vi "CreatingandAccessingFiles.vi"() -> ()   [LabVIEW 2020]
panel:
  out "appended path":path
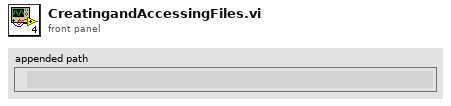
[diagram p1: front panel]
types:
  T1 = enum16{"open", "replace", "create", "open or create", "replace or create", "replace or create with confirmation"}
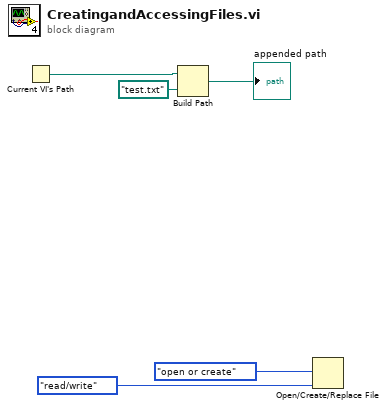
[diagram p0: block diagram]
diagram:
  n1 = Current VI's Path() -> (path=w1:path)
  n2 = Build Path(base path=w1, name or relative path=path "test.txt") -> (appended path=→"appended path":path)
  n3 = Open/Create/Replace File(operation (0:open)=T1."open or create", access (0:read/write)=enum16{"read/write", "read-only", "write-only"}."read/write") -> ()  [unwired: 4 in, 3 out]
